vi "4.6.（3）.vi"() -> ()   [LabVIEW 2017]
panel:
  in  "停止":bool
  out "和":dbl
  in  "加数2":dbl
  in  "加数1":dbl
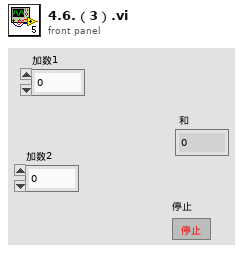
[diagram p1: front panel]
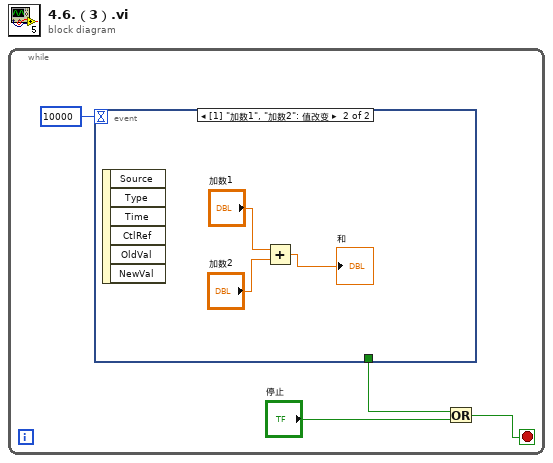
[diagram p0: block diagram]
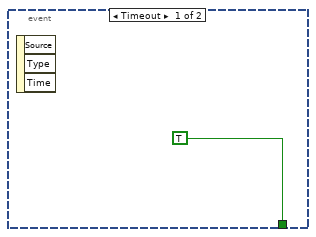
[diagram p2: hidden frame]
diagram:
  n1 = while {
    stop <- w2 stop-if-true
    n2 = event shown="[1] \"加数1\", \"加数2\": 值改变" {
      selector: _ -> [_ _]
      dyn-events: _ -> [_ _]
      timeout: 10000 -> [_ _]
      tunnel: [TRUE _] -> w3
      event Timeout {
        n3 = event-data() -> ()  [unwired: 1 in, 3 out]
      }
      event "加数1", "加数2": Value Change {
        n4 = event-data() -> ()  [unwired: 1 in, 6 out]
        n5 = Add(x="加数1", y="加数2") -> (x+y=→"和":dbl)
      }
    }
    n6 = Or(x=w3, y="停止") -> (x .or. y?=w2:bool)
  }
